vi "PH_Sequencer.PC _PHELIXStatus.vi"(0 "i ref in":refnum<vi>, 2 "Tagname":string, 3 "Tagvalue":T1=4 caption="Enabling State" items=["no info", "off/false", "on/true", "Failure", "Alarm"], 5 "error in (no error)":errorcluster) -> (14 "i ref out":refnum<vi>, 19 "error out":errorcluster)   [LabVIEW 2009]
doc: "This VI writes the incoming information for Emergency off, Laser-, PreAmp- and MainAmp-Freigabe to the related GUI element and to own attributes."
uses:
  PH_Sequencer.lvlib
  PH_Common/Ctrls/Device State.ctl
  PH_Common/Ctrls/Enabling State.ctl
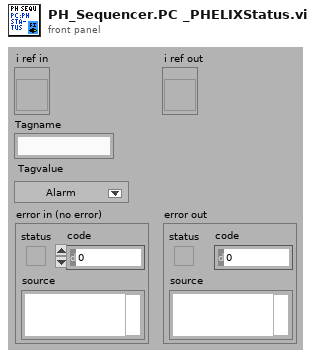
[diagram p1: front panel]
types:
  T1 = typedef "Device State.ctl" = i32
  T2 = typedef "PH_Sequencer.lvlib/PH_Sequencer.i attribute.ctl" = cluster{"GUI Refs":cluster{"Main Off":refnum<vi>, "Fire":refnum<vi>, "Status":refnum<vi>, "Ready":refnum<vi>, "Waiting Time":refnum<vi>, "Timeout":refnum<vi>, "SMs ok":refnum<vi>, "PP DP Ready":refnum<vi>, "Sequencer SM State":refnum<vi>, "PP PA Ready":refnum<vi>, "Calorimeter":refnum<vi>, "Beamline Ready":refnum<vi>, "Clear Beamline":refnum<vi>, "Linkage PPMA Rods":refnum<vi>, "Linkage Current PA":refnum<vi>, "Linkage Current MA":refnum<vi>, "Linkage PPMA Rods 2":refnum<vi>, "Linkage PPMA Rods 3":refnum<vi>, "Linkage Current MA 2":refnum<vi>, "Linkage Current MA 3":refnum<vi>, "PP Booster Ready":refnum<vi>, "PP FR Ready":refnum<vi>, "Timing Ready":refnum<vi>, "State Timing":refnum<vi>, "Force Timing":refnum<vi>, "PSDB Shot Comment":refnum<vi>, "State PA Backreflection":refnum<vi>, "Beamline Z6 Ready":refnum<vi>, "Clear Z6 Beamline":refnum<vi>, "Sequence length":refnum<vi>, "Timing Mode":refnum<vi>, "Slow Trigger Settings":refnum<vi>, "Experiment Description":refnum<vi>, "State PSDB":refnum<vi>, "PSDB Ready":refnum<vi>, "Set PSDB Settings":refnum<vi>, "Get PSDB Info":refnum<vi>, "Take Snapshot":refnum<vi>, "Shottype":refnum<vi>, "Experiment":refnum<vi>, "PA Energy":refnum<vi>, "MA Energy":refnum<vi>, "MA Gain":refnum<vi>}, "Status Info":cluster{"Machine Status":T3, "WaitingTime":i32, "Timeout":bool}, "Readyness":cluster{"Ready to shot":bool, "PP DP Ready":bool, "PPPA Ready":bool, "BL Ready":bool, "PP Booster Ready":bool, "PP FR Ready":bool, "Timing Ready":bool, "BL Z6 Ready":bool, "PSDBReady":bool}, "Instancenames":cluster{"PPMA Rods":string, "PP Current Meas":string, "Beamline":string, "PA Backrefl Meas":string, "Beamline Z6":string}, "Data to read":bool, "Calorimeter":cluster{"Instancename":string, "On":bool, "linked":bool}, "Linkage":cluster{"PPMA Rods":bool, "PP Current Meas":bool, "Beamline":bool, "PA Backrefl Meas":bool, "Beamline Z6":bool}, "PU Info":T4[], "HV Info":T5[], "PSU Info":T6[], "Refs PU on":refnum<vi>[], "Refs Set Voltage PU":refnum<vi>[], "Refs State PU":refnum<vi>[], "Refs State SM PU":refnum<vi>[], "Refs Waiting Time PU":refnum<vi>[], "Refs TO SM PU":refnum<vi>[], "Refs Voltage PU":refnum<vi>[], "Timing":cluster{"Instance":string, "linked":bool, "Status":T3, "Timing Mode":T7, "Slow Trigger Settings":T8, "Info available":cluster{"ext SlowTrigger":bool, "T2":bool, "Mode":bool, "Delay Slow Trigger":bool}}, "GUI Manager Path":string, "Service ID R2S":i32, "PSDB":cluster{"Controller Instance":string, "Controller Status":T3, "Controller linked":bool, "Settings acknowledged":bool, "Current Experiment ID":i16, "Current Shot Type":i16, "Current Comment":string, "Remember Settings":bool, "Write 2 early":bool}, "PSDB Data":cluster{"Main Off?":bool, "Sequence Length":dbl, "Sequence startet":timestamp}, "Beamline":refnum<vi>[], "Powermeter":cluster{"PA":cluster{"Instance":string, "Energy [J]":dbl, "in use":bool}, "MA":cluster{"Instance":string, "Energy [J]":dbl, "in use":bool}, "MA Gain":dbl}}
  T3 = typedef "Status.ctl" = i16
  T4 = typedef "PH_Sequencer.lvlib/PH_Sequencer.PU Info.ctl" = cluster{"Instancename":string, "PU on":bool, "State":T3, "Waiting time":i32, "Set Voltage":dbl, "State SM":string, "Timeout SM":string, "linked":bool}
  T5 = typedef "PH_Sequencer.lvlib/PH_Sequencer.HV Meas Info.ctl" = cluster{"Instancename":string, "linked":bool, "Tagname Meas Voltage":string}
  T6 = typedef "PH_Sequencer.lvlib/PH_Sequencer.PSU Info.ctl" = cluster{"Instancename":string, "linked":bool, "Tagname Applied Voltage":string}
  T7 = typedef "PH_Timing.lvlib/PH_Timing.Timing Mode.ctl" = cluster{"T2 [s]":i16, "Modeselector":enum32{"10 Hz", "0.5 Hz", "Shot"}}
  T8 = typedef "PH_Timing.lvlib/PH_Timing.Slow Trigger Settings.ctl" = cluster{"Delay [ms]":dbl, "externally triggered?":bool}
  T9 = cluster{"DIM Service Name":string, "GUI Ref":refnum<vi>, "State":enum16{"no info", "off/false", "Alarm"}}
  T10 = cluster{"DIM Service Name":bool, "GUI Ref":bool, "State":bool}
  T11 = typedef "Enabling State.ctl" = i32
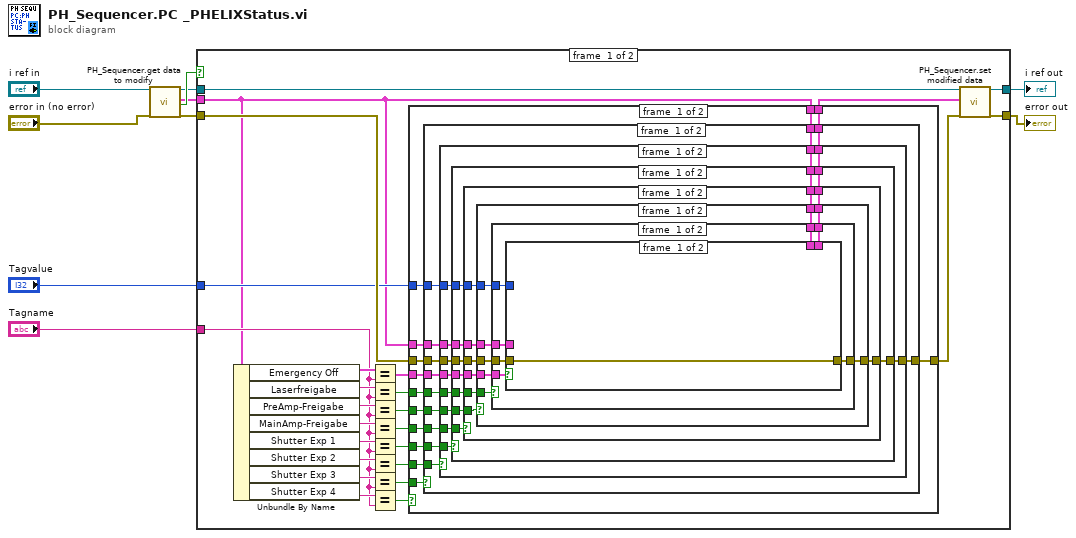
[diagram p0: block diagram]
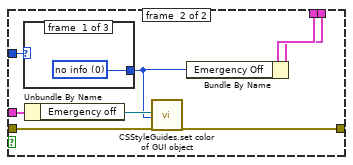
[diagram p2: hidden frame]
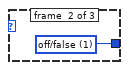
[diagram p3: hidden frame]
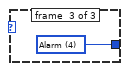
[diagram p4: hidden frame]
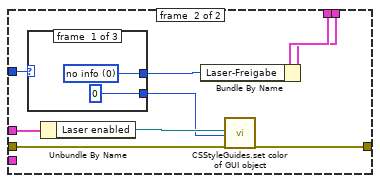
[diagram p5: hidden frame]
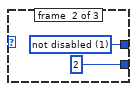
[diagram p6: hidden frame]
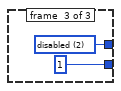
[diagram p7: hidden frame]
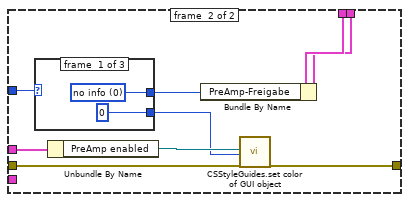
[diagram p8: hidden frame]
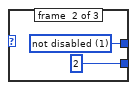
[diagram p9: hidden frame]
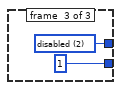
[diagram p10: hidden frame]
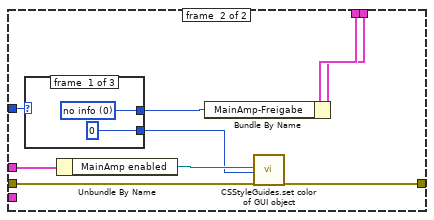
[diagram p11: hidden frame]
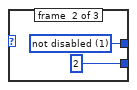
[diagram p12: hidden frame]
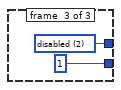
[diagram p13: hidden frame]
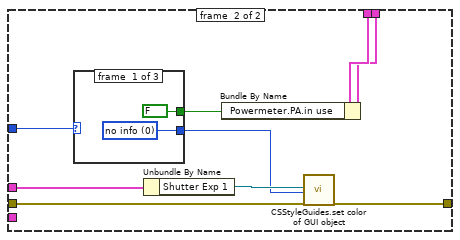
[diagram p14: hidden frame]
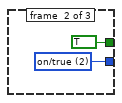
[diagram p15: hidden frame]
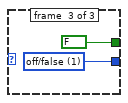
[diagram p16: hidden frame]
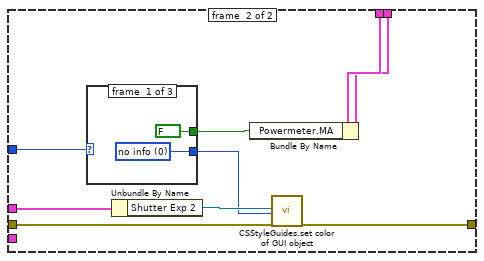
[diagram p17: hidden frame]
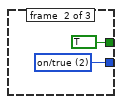
[diagram p18: hidden frame]
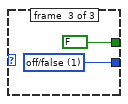
[diagram p19: hidden frame]
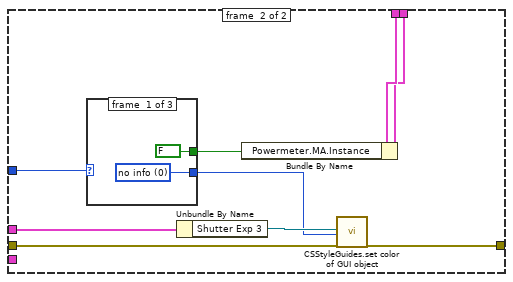
[diagram p20: hidden frame]
diagram:
  n1 = call "PH_Sequencer.get data to modify.vi"("i ref in"="i ref in", "error in (no error)"="error in (no error)") -> ("i ref out"=w5:refnum<vi>, "i attribute"=w9:T2, "timed out"=w10:bool, "error out"=w7:errorcluster)  [unwired: 14 in]
  n2 = case shown="False" w10 {
    tunnel: w5 -> [w35 w225]
    tunnel: [w34 w225] -> w6
    tunnel: w7 -> [w24 w224]
    tunnel: [w33 w224] -> w8
    tunnel: w9 -> [w11 _]
    tunnel: "Tagvalue" -> [w21 _]
    tunnel: "Tagname" -> [w16 _]
    frame #0 {
      n3 = Unbundle By Name(w11) -> ("Emergency Off"=w29:T9, "Laserfreigabe"=w28:string, "PreAmp-Freigabe"=w30:string, "MainAmp-Freigabe"=w32:string, "Shutter Exp 1"=w20:string, "Shutter Exp 2"=w19:string, "Shutter Exp 3"=w18:string, "Shutter Exp 4"=w17:string)
      n4 = Equal?(x=w29, y=w16) -> (x = y?=w25:T10)
      n5 = Equal?(x=w28, y=w16) -> (x = y?=w26:bool)
      n6 = Equal?(x=w30, y=w16) -> (x = y?=w27:bool)
      n7 = Equal?(x=w32, y=w16) -> (x = y?=w31:bool)
      n8 = Equal?(x=w20, y=w16) -> (x = y?=w15:bool)
      n9 = Equal?(x=w19, y=w16) -> (x = y?=w14:bool)
      n10 = Equal?(x=w18, y=w16) -> (x = y?=w13:bool)
      n11 = Equal?(x=w17, y=w16) -> (x = y?=w12:bool)
      n12 = case shown="False" w12 {
        tunnel: w31 -> [w48 _]
        tunnel: w27 -> [w47 _]
        tunnel: w26 -> [w46 _]
        tunnel: w25 -> [w45 _]
        tunnel: w24 -> [w44 w215]
        tunnel: [w43 w214] -> w23
        tunnel: w11 -> [w42 w217]
        tunnel: [w41 w210] -> w22
        tunnel: w21 -> [w40 w213]
        tunnel: w15 -> [w39 _]
        tunnel: w14 -> [w38 _]
        tunnel: w13 -> [w37 _]
        tunnel: w11 -> [w36 w211]
        frame #0 {
          n13 = case shown="False" w37 {
            tunnel: w48 -> [w60 _]
            tunnel: w47 -> [w59 _]
            tunnel: w46 -> [w58 _]
            tunnel: w45 -> [w57 _]
            tunnel: w44 -> [w56 w199]
            tunnel: [w55 w198] -> w43
            tunnel: w42 -> [w54 w200]
            tunnel: [w53 w195] -> w41
            tunnel: w40 -> [w52 w197]
            tunnel: w39 -> [w51 _]
            tunnel: w38 -> [w50 _]
            tunnel: w36 -> [w49 w202]
            frame #0 {
              n14 = case shown="False" w50 {
                tunnel: w60 -> [w71 _]
                tunnel: w59 -> [w70 _]
                tunnel: w58 -> [w69 _]
                tunnel: w57 -> [w68 _]
                tunnel: w56 -> [w67 w184]
                tunnel: [w66 w183] -> w55
                tunnel: w54 -> [w65 w185]
                tunnel: [w64 w180] -> w53
                tunnel: w52 -> [w63 w182]
                tunnel: w51 -> [w62 _]
                tunnel: w49 -> [w61 w187]
                frame #0 {
                  n15 = case shown="False" w62 {
                    tunnel: w71 -> [w81 _]
                    tunnel: w70 -> [w80 _]
                    tunnel: w69 -> [w79 _]
                    tunnel: w68 -> [w78 _]
                    tunnel: w67 -> [w77 w169]
                    tunnel: [w76 w168] -> w66
                    tunnel: w65 -> [w75 w170]
                    tunnel: [w74 w165] -> w64
                    tunnel: w63 -> [w73 w167]
                    tunnel: w61 -> [w72 w172]
                    frame #0 {
                      n16 = case shown="False" w81 {
                        tunnel: w80 -> [w90 _]
                        tunnel: w79 -> [w89 _]
                        tunnel: w78 -> [w88 _]
                        tunnel: w75 -> [w87 w151]
                        tunnel: w77 -> [w86 w154]
                        tunnel: [w85 w155] -> w76
                        tunnel: w72 -> [w84 w153]
                        tunnel: [w83 w152] -> w74
                        tunnel: w73 -> [w82 w150]
                        frame #0 {
                          n17 = case shown="False" w90 {
                            tunnel: w89 -> [w98 _]
                            tunnel: w88 -> [w97 _]
                            tunnel: w87 -> [w96 w135]
                            tunnel: w86 -> [w95 w139]
                            tunnel: [w94 w140] -> w85
                            tunnel: w84 -> [w93 w138]
                            tunnel: [w92 w137] -> w83
                            tunnel: w82 -> [w91 w136]
                            frame #0 {
                              n18 = case shown="True" w98 {
                                tunnel: w97 -> [w105 _]
                                tunnel: w96 -> [w104 w122]
                                tunnel: w95 -> [w103 w123]
                                tunnel: [w102 w124] -> w94
                                tunnel: w93 -> [w101 w126]
                                tunnel: [w100 w125] -> w92
                                tunnel: w91 -> [w99 w121]
                                frame #0 {
                                n19 = case shown="True" w105 {
                                tunnel: w104 -> [_ w115]
                                tunnel: w103 -> [w107 w113]
                                tunnel: [w107 w112] -> w102
                                tunnel: w101 -> [w106 w111]
                                tunnel: [w106 w110] -> w100
                                tunnel: w99 -> [_ w109]
                                frame #0 {
                                }
                                frame #1 {
                                n20 = case shown="2" w109 {
                                tunnel: [w116 w117 w118] -> w108
                                frame #0 {
                                w116 = T1 0 items=["no info", "off/false", "on/true", "Failure", "Alarm"] ("Status Info.Emergency Off")
                                }
                                frame #1 {
                                w117 = T1 1 items=["no info", "off/false", "on/true", "Failure", "Alarm"] ("Status Info.Emergency Off")
                                }
                                frame #2 {
                                w118 = T1 4 items=["no info", "off/false", "on/true", "Failure", "Alarm"] ("Status Info.Emergency Off")
                                }
                                }
                                n21 = Unbundle By Name(w115) -> ("Emergency off"=w114:refnum<vi>)
                                n22 = call "CSStyleGuides.set color of GUI object.vi"("GUI object Ref"=w114, "State"=w108, "error in (no error)"=w113) -> ("error out"=w112:errorcluster)  [unwired: 16 in]
                                n23 = Bundle By Name(cluster=w111, "Emergency Off"=w108) -> (w110:T2)
                                }
                                }
                                }
                                frame #1 {
                                n24 = case shown="1" w121 {
                                tunnel: [w129 w131 w133] -> w120
                                tunnel: [0 2 1] -> w119
                                frame #0 {
                                w129 = T11 0 items=["no info", "not disabled", "disabled"] ("Status Info.Laser-Freigabe")
                                }
                                frame #1 {
                                w131 = T11 1 items=["no info", "not disabled", "disabled"] ("Status Info.Laser-Freigabe")
                                }
                                frame #2 {
                                w133 = T11 2 items=["no info", "not disabled", "disabled"] ("Status Info.Laser-Freigabe")
                                }
                                }
                                n25 = Unbundle By Name(w122) -> ("Laser enabled"=w127:refnum<vi>)
                                n26 = Bundle By Name(cluster=w126, "Laser-Freigabe"=w120) -> (w125:T2)
                                n27 = call "CSStyleGuides.set color of GUI object.vi"("GUI object Ref"=w127, "State"=w119, "error in (no error)"=w123) -> ("error out"=w124:errorcluster)  [unwired: 16 in]
                                }
                              }
                            }
                            frame #1 {
                              n28 = case shown="2" w136 {
                                tunnel: [w144 w146 w148] -> w134
                                tunnel: [0 2 1] -> w141
                                frame #0 {
                                w144 = T11 0 items=["no info", "not disabled", "disabled"] ("Status Info.Laser-Freigabe")
                                }
                                frame #1 {
                                w146 = T11 1 items=["no info", "not disabled", "disabled"] ("Status Info.Laser-Freigabe")
                                }
                                frame #2 {
                                w148 = T11 2 items=["no info", "not disabled", "disabled"] ("Status Info.Laser-Freigabe")
                                }
                              }
                              n29 = Unbundle By Name(w135) -> ("PreAmp enabled"=w142:refnum<vi>)
                              n30 = Bundle By Name(cluster=w138, "PreAmp-Freigabe"=w134) -> (w137:T2)
                              n31 = call "CSStyleGuides.set color of GUI object.vi"("GUI object Ref"=w142, "State"=w141, "error in (no error)"=w139) -> ("error out"=w140:errorcluster)  [unwired: 16 in]
                            }
                          }
                        }
                        frame #1 {
                          n32 = case shown="2" w150 {
                            tunnel: [w159 w161 w163] -> w149
                            tunnel: [0 2 1] -> w156
                            frame #0 {
                              w159 = T11 0 items=["no info", "not disabled", "disabled"] ("Status Info.Laser-Freigabe")
                            }
                            frame #1 {
                              w161 = T11 1 items=["no info", "not disabled", "disabled"] ("Status Info.Laser-Freigabe")
                            }
                            frame #2 {
                              w163 = T11 2 items=["no info", "not disabled", "disabled"] ("Status Info.Laser-Freigabe")
                            }
                          }
                          n33 = Unbundle By Name(w151) -> ("MainAmp enabled"=w157:refnum<vi>)
                          n34 = Bundle By Name(cluster=w153, "MainAmp-Freigabe"=w149) -> (w152:T2)
                          n35 = call "CSStyleGuides.set color of GUI object.vi"("GUI object Ref"=w157, "State"=w156, "error in (no error)"=w154) -> ("error out"=w155:errorcluster)  [unwired: 16 in]
                        }
                      }
                    }
                    frame #1 {
                      n36 = case shown="1" w167 {
                        tunnel: [w174 w176 w178] -> w166
                        tunnel: [FALSE TRUE FALSE] -> w164
                        frame #0 {
                          w174 = T1 0 items=["no info", "off/false", "on/true", "Failure", "Alarm"] ("Status Info.Emergency Off")
                        }
                        frame #1 {
                          w176 = T1 2 items=["no info", "off/false", "on/true", "Failure", "Alarm"] ("Status Info.Emergency Off")
                        }
                        frame #2 {
                          w178 = T1 1 items=["no info", "off/false", "on/true", "Failure", "Alarm"] ("Status Info.Emergency Off")
                        }
                      }
                      n37 = Unbundle By Name(w170) -> ("Shutter Exp 1"=w171:refnum<vi>)
                      n38 = Bundle By Name(cluster=w172, "Powermeter.PA.in use"=w164) -> (w165:T2)
                      n39 = call "CSStyleGuides.set color of GUI object.vi"("GUI object Ref"=w171, "State"=w166, "error in (no error)"=w169) -> ("error out"=w168:errorcluster)  [unwired: 16 in]
                    }
                  }
                }
                frame #1 {
                  n40 = case shown="1" w182 {
                    tunnel: [w189 w191 w193] -> w181
                    tunnel: [FALSE TRUE FALSE] -> w179
                    frame #0 {
                      w189 = T1 0 items=["no info", "off/false", "on/true", "Failure", "Alarm"] ("Status Info.Emergency Off")
                    }
                    frame #1 {
                      w191 = T1 2 items=["no info", "off/false", "on/true", "Failure", "Alarm"] ("Status Info.Emergency Off")
                    }
                    frame #2 {
                      w193 = T1 1 items=["no info", "off/false", "on/true", "Failure", "Alarm"] ("Status Info.Emergency Off")
                    }
                  }
                  n41 = Unbundle By Name(w185) -> ("Shutter Exp 2"=w186:refnum<vi>)
                  n42 = Bundle By Name(cluster=w187, "Powermeter.MA"=w179) -> (w180:T2)
                  n43 = call "CSStyleGuides.set color of GUI object.vi"("GUI object Ref"=w186, "State"=w181, "error in (no error)"=w184) -> ("error out"=w183:errorcluster)  [unwired: 16 in]
                }
              }
            }
            frame #1 {
              n44 = case shown="1" w197 {
                tunnel: [w204 w206 w208] -> w196
                tunnel: [FALSE TRUE FALSE] -> w194
                frame #0 {
                  w204 = T1 0 items=["no info", "off/false", "on/true", "Failure", "Alarm"] ("Status Info.Emergency Off")
                }
                frame #1 {
                  w206 = T1 2 items=["no info", "off/false", "on/true", "Failure", "Alarm"] ("Status Info.Emergency Off")
                }
                frame #2 {
                  w208 = T1 1 items=["no info", "off/false", "on/true", "Failure", "Alarm"] ("Status Info.Emergency Off")
                }
              }
              n45 = Unbundle By Name(w200) -> ("Shutter Exp 3"=w201:refnum<vi>)
              n46 = Bundle By Name(cluster=w202, "Powermeter.MA.Instance"=w194) -> (w195:T2)
              n47 = call "CSStyleGuides.set color of GUI object.vi"("GUI object Ref"=w201, "State"=w196, "error in (no error)"=w199) -> ("error out"=w198:errorcluster)  [unwired: 16 in]
            }
          }
        }
        frame #1 {
          n48 = case shown="1" w213 {
            tunnel: [w219 w221 w223] -> w212
            tunnel: [FALSE TRUE FALSE] -> w209
            frame #0 {
              w219 = T1 0 items=["no info", "off/false", "on/true", "Failure", "Alarm"] ("Status Info.Emergency Off")
            }
            frame #1 {
              w221 = T1 2 items=["no info", "off/false", "on/true", "Failure", "Alarm"] ("Status Info.Emergency Off")
            }
            frame #2 {
              w223 = T1 1 items=["no info", "off/false", "on/true", "Failure", "Alarm"] ("Status Info.Emergency Off")
            }
          }
          n49 = Unbundle By Name(w217) -> ("Shutter Exp 4"=w216:refnum<vi>)
          n50 = Bundle By Name(cluster=w211, "Powermeter.MA.Energy [J]"=w209) -> (w210:T2)
          n51 = call "CSStyleGuides.set color of GUI object.vi"("GUI object Ref"=w216, "State"=w212, "error in (no error)"=w215) -> ("error out"=w214:errorcluster)  [unwired: 16 in]
        }
      }
      n52 = call "PH_Sequencer.set modified data.vi"("i ref in"=w35, "i attribute"=w22, "error in (no error)"=w23) -> ("i ref out"=w34:refnum<vi>, "error out"=w33:errorcluster)  [unwired: 15 in]
    }
    frame #1 {
    }
  }
  "error out" <- w8
  "i ref out" <- w6
